vi "校准设置页.vi"() -> ()   [LabVIEW 2016, in "斯坦道总磷.lvlib"]
uses:
  <vilib>/ptbypt/NI_PtbyPt.lvlib
panel:
  in  "校准任务":bool
  in  "历史数据导入":T1(radio)
  out "刷新时间":string
  out "模型刷新":bool
  in  "校准按钮":T1(radio)
  in  "仪器写入":bool
  in  "辅助计算":bool
  in  "曲线模型":T2={"标液浓度1"=0.0, "测量吸光度1"=0.0, "样品1启用"=FALSE, "标液浓度2"=0.0, "测量吸光度2"=0.0, "样品2启用"=FALSE, "标液浓度3"=0.0, "测量吸光度3"=0.0, "样品3启用"=FALSE, "标液浓度4"=0.0, "测量吸光度4"=0.0, "样品4启用"=FALSE, "标液浓度5"=0.0, "测量吸光度5"=0.0, "样品5启用"=FALSE, "模型"=enum."线性", "精度"=4.0, "XY图"=[], "拟合公式"="", "r^2"=0.0, "标样一校准时间"=timestamp(0 s since 1904-01-01), "标样二校准时间"=timestamp(0 s since 1904-01-01), "标样三校准时间"=timestamp(0 s since 1904-01-01), "标样四校准时间"=timestamp(0 s since 1904-01-01), "标样五校准时间"=timestamp(0 s since 1904-01-01), "二次方程"={"c"=0.0, "x"=0.0, "x^2"=0.0}, "标定时间"=timestamp(0 s since 1904-01-01)} {"标定时间" format="%<%y/%m/%d %H:%M:%S>T"; "标样五校准时间" format="%<%y/%m/%d %H:%M:%S>T"; "标样四校准时间" format="%<%y/%m/%d %H:%M:%S>T"; "标样三校准时间" format="%<%y/%m/%d %H:%M:%S>T"; "标样二校准时间" format="%<%y/%m/%d %H:%M:%S>T"; "标样一校准时间" format="%<%y/%m/%d %H:%M:%S>T"; "r^2" format="%.7f"; "测量吸光度5" format="%#.6f"; "测量吸光度4" format="%#.6f"; "测量吸光度3" format="%#.6f"; "测量吸光度2" format="%#.6f"; "测量吸光度1" format="%#.6f"}
  in  "测量模式":T3(ring)
  in  "参数下拉列表":u16(ring)
  in  "量程下拉列表":enum16{"低量程", "高量程"}(ring)
  # "校准时间"
  # "标液浓度"
  # "吸光值"
  # "空白"
  # "标样一"
  # "标样二"
  # "零点"
  # "跨度"
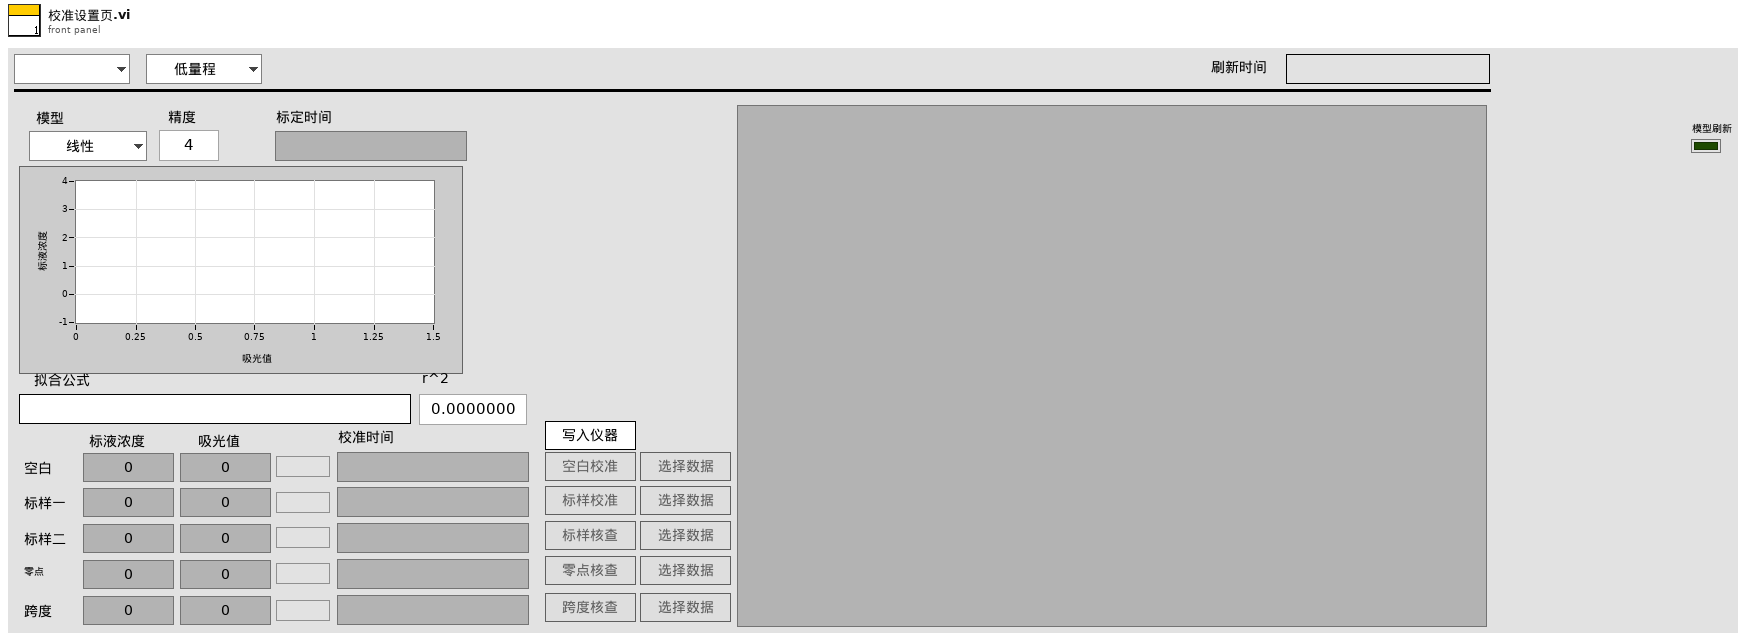
[diagram p1: front panel]
types:
  T1 = enum32{"未选择", "空白校准", "标样校准", "标样核查", "零点核查", "跨度核查"}
  T2 = cluster{"标液浓度1":dbl, "测量吸光度1":dbl, "样品1启用":bool, "标液浓度2":dbl, "测量吸光度2":dbl, "样品2启用":bool, "标液浓度3":dbl, "测量吸光度3":dbl, "样品3启用":bool, "标液浓度4":dbl, "测量吸光度4":dbl, "样品4启用":bool, "标液浓度5":dbl, "测量吸光度5":dbl, "样品5启用":bool, "模型":enum32{"线性", "多项式"}, "精度":dbl, "XY图":cluster{"X Values":dbl[], "Y Values":dbl[]}[], "拟合公式":string, "r^2":dbl, "标样一校准时间":timestamp, "标样二校准时间":timestamp, "标样三校准时间":timestamp, "标样四校准时间":timestamp, "标样五校准时间":timestamp, "二次方程":cluster{"c":dbl, "x":dbl, "x^2":dbl}, "标定时间":timestamp}
  T3 = enum16{"跨度核查", "水样测量", "零点核查", "标样核查", "加标回收", "快捷测试", "空白校准", "标样校准"}
  T4 = typedef "斯坦道总磷.lvlib/校准任务.ctl" = cluster{"id":u16, "任务类型":enum16{"未选择", "空白校准", "标样校准", "标样核查", "零点核查", "跨度核查"}, "量程下拉列表":enum16{"低量程", "高量程"}, "状态":enum16{"已执行", "待执行", "执行中", "停止"}, "标液浓度":dbl, "吸光值":dbl, "校准时间":timestamp}
  T5 = enum8{"Enabled", "Disabled", "Disabled and Grayed Out"}
  T6 = typedef "LVStringsAndValuesArrayTypeDef_U16.ctl" = cluster{"String":string, "Value":u16}[]
  T7 = cluster{"标液浓度1":dbl, "测量吸光度1":dbl, "样品1启用":bool, "标液浓度2":dbl, "测量吸光度2":dbl, "样品2启用":bool, "标液浓度3":dbl, "测量吸光度3":dbl, "样品3启用":bool, "标液浓度4":dbl, "测量吸光度4":dbl, "样品4启用":bool, "标液浓度5":dbl, "测量吸光度5":dbl, "样品5启用":bool, "模型":enum32{"线性", "多项式"}, "精度":dbl, "XY图":cluster{"X Values":dbl[], "Y Values":dbl[]}[], "拟合公式":string, "r^2":dbl, "标样一校准时间":timestamp, "标样二校准时间":timestamp, "标样三校准时间":timestamp, "标样四校准时间":timestamp, "标样五校准时间":timestamp, "二次方程":cluster{"c":dbl, "x":dbl, "x^2":dbl}, "标定时间":timestamp}[]
  T8 = cluster{"时间":timestamp, "标液值":dbl, "检测值":dbl, "吸光值":dbl}
  T9 = enum32{"Bad", "Idle", "Run top level", "Running"}
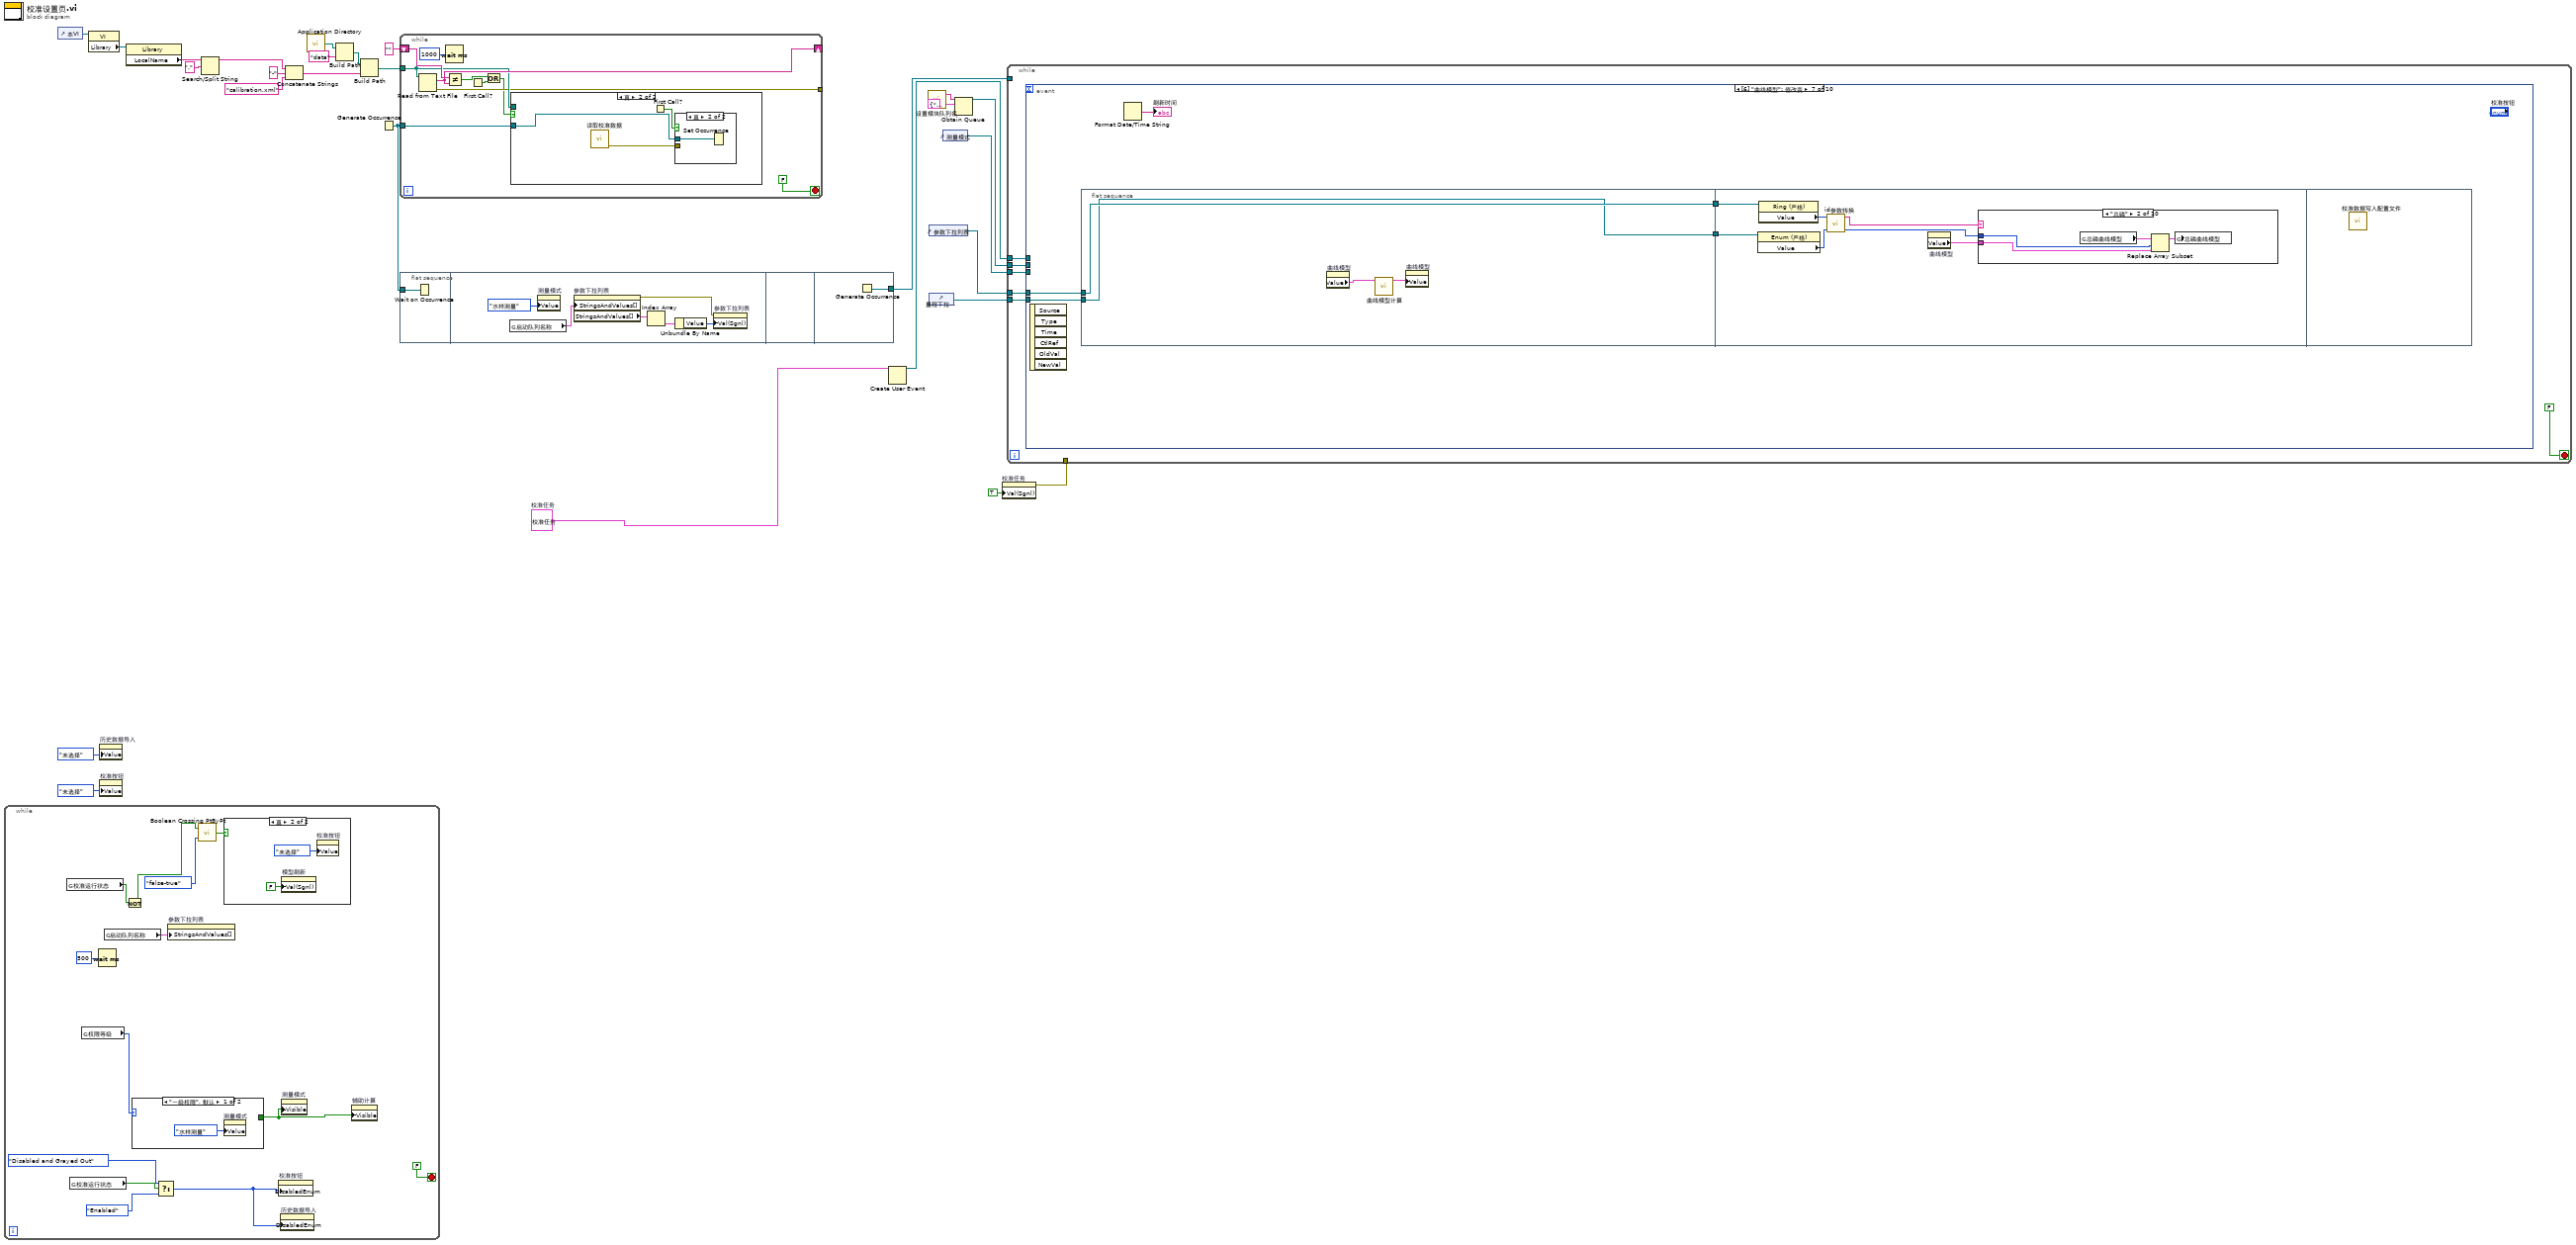
[diagram p0: block diagram]
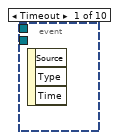
[diagram p4: hidden frame]
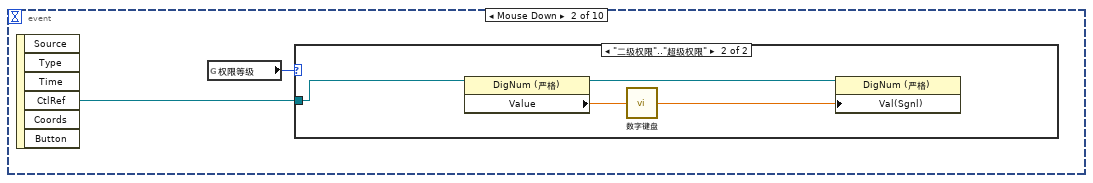
[diagram p5: hidden frame]
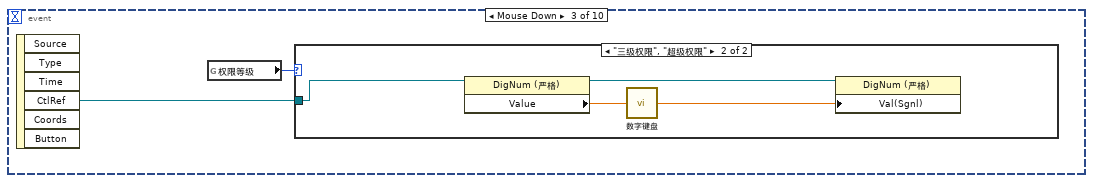
[diagram p7: hidden frame]
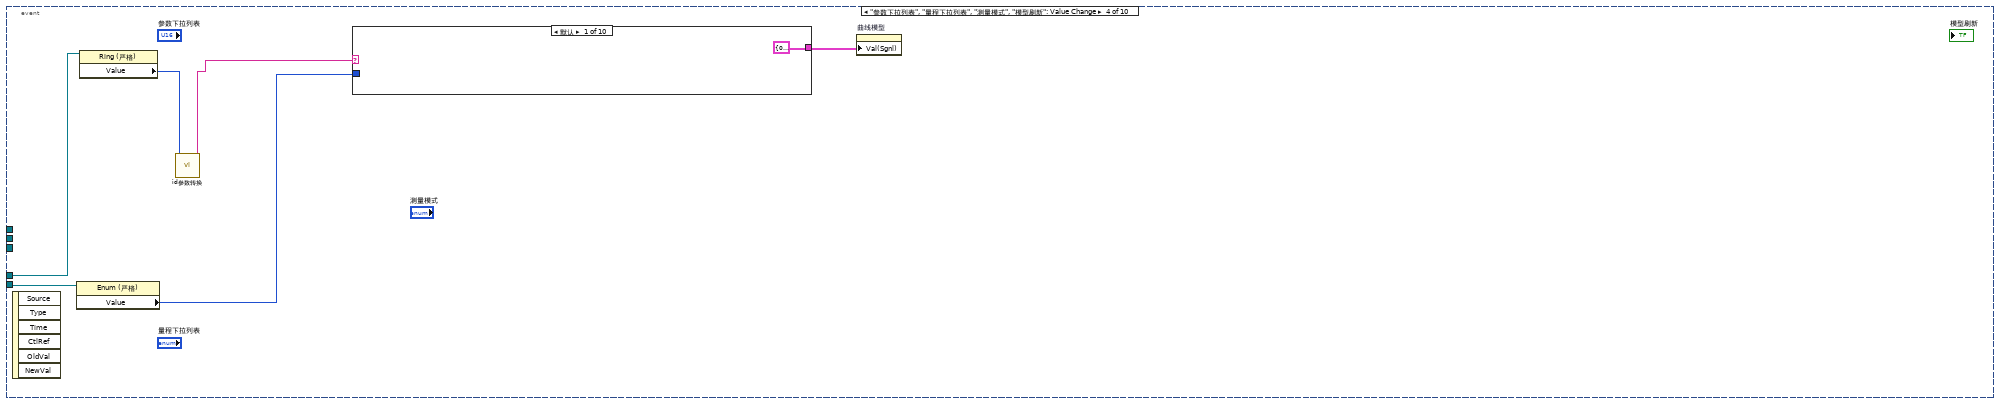
[diagram p9: hidden frame]
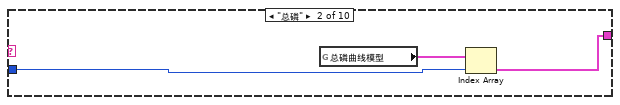
[diagram p10: hidden frame]
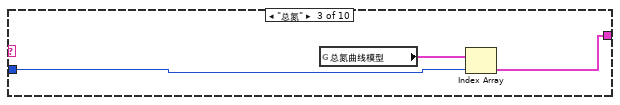
[diagram p11: hidden frame]
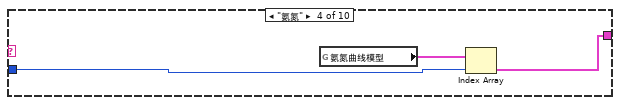
[diagram p12: hidden frame]
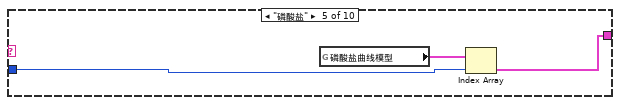
[diagram p13: hidden frame]
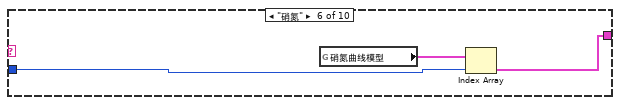
[diagram p14: hidden frame]
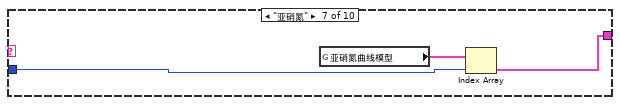
[diagram p15: hidden frame]
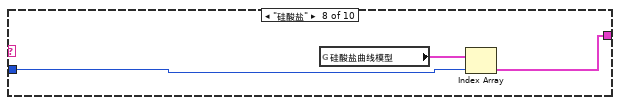
[diagram p16: hidden frame]
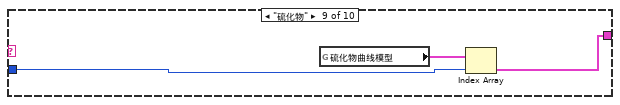
[diagram p17: hidden frame]
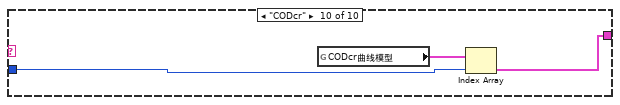
[diagram p18: hidden frame]
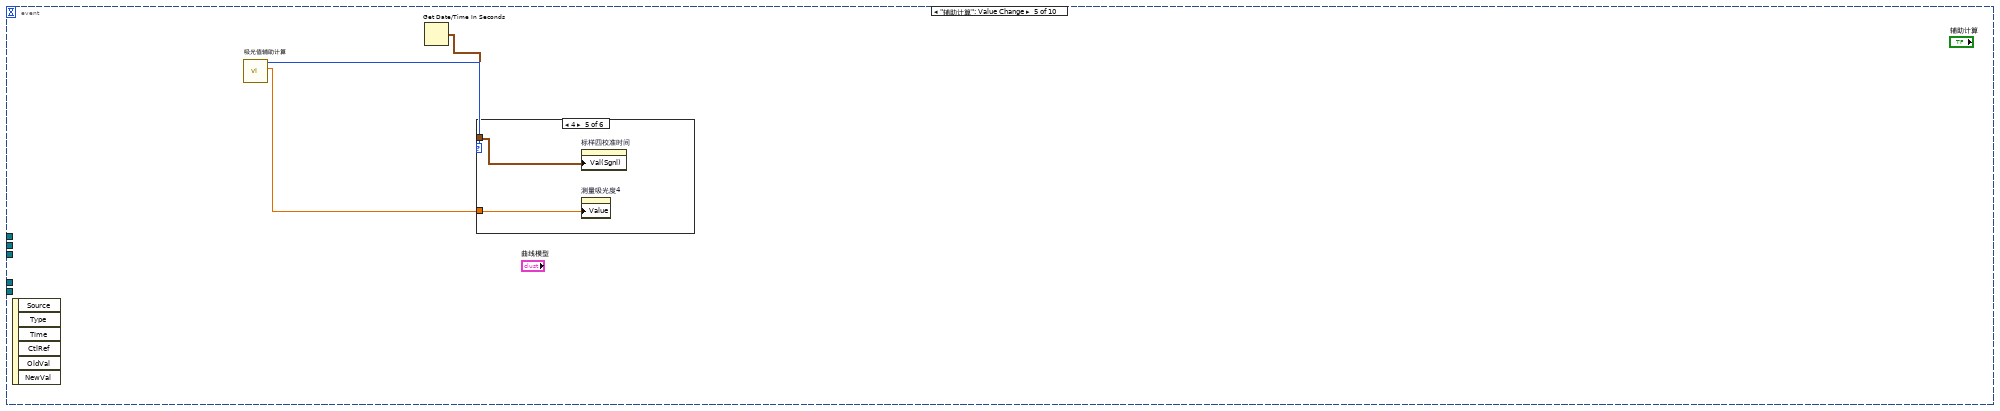
[diagram p19: hidden frame]
diagram:
  w3 = T4 {"id"=1, "任务类型"=enum."未选择", "量程下拉列表"=enum."低量程", "状态"=enum."已执行", "标液浓度"=0.0, "吸光值"=0.0, "校准时间"=timestamp(0 s since 1904-01-01)}  # 校准任务
  n1 = while {
    stop <- FALSE stop-if-true
    n2 = global read "VAR总磷总氮全局变量.vi" "校准运行状态"() -> (w34:bool)
    n3 = global read "VAR总磷总氮全局变量.vi" "校准运行状态"() -> (w31:bool)
    n4 = global read "VAR总磷总氮全局变量.vi" "权限等级"() -> (w38:enum16{"一级权限", "二级权限", "三级权限", "超级权限"})
    n5 = Wait (ms)(milliseconds to wait=u32 500 ("等待时间（毫秒）")) -> ()  [unwired: 1 out]
    n6 = global read "总磷总氮断电保存全局变量.vi" "启动队列名称"() -> (w35:cluster{"String":string, "Value":u16}[])
    n7 = Not(x=w34) -> (.not. x?=w33:bool)
    n8 = case shown="\"一级权限\", 默认" w38 {
      tunnel: [_ TRUE ("可见")] -> w32
      frame "一级权限", Default {
        n9 = property on="测量模式" class="Enum (严格)"("Value"=T3."水样测量" ("测量模式")) -> ()  [unwired: 2 in, 2 out]
      }
      frame "三级权限", "超级权限" {
      }
    }
    n10 = Select(t=T5."Disabled and Grayed Out" ("禁用"), s=w31, f=T5."Enabled" ("禁用")) -> (s? t:f=w29:T5)
    n11 = property on="参数下拉列表" class="Ring (严格)"("StringsAndValues[]"=w35) -> ()  [unwired: 2 in, 2 out]
    n12 = call <vilib>:"Boolean Crossing PtByPt.vi"("direction"=enum16{"either", "false-true", "true-false"}."false-true", "input"=w33) -> ("crossing"=w36:bool)  [unwired: 1 in]
    n13 = case shown="真" w36 {
      frame False {
      }
      frame True {
        n14 = property on="模型刷新" class="Bool (严格)"("Val(Sgnl)"=FALSE ("值(信号)")) -> ()  [unwired: 2 in, 2 out]
        n15 = property on="校准按钮" class="RadioBtnsControl (严格)"("Value"=T1."未选择" ("校准按钮")) -> ()  [unwired: 2 in, 2 out]
      }
    }
    n16 = property on="校准按钮" class="RadioBtnsControl (严格)"("DisabledEnum"=w29) -> ()  [unwired: 2 in, 2 out]
    n17 = property on="历史数据导入" class="RadioBtnsControl (严格)"("DisabledEnum"=w29) -> ()  [unwired: 2 in, 2 out]
    n18 = property on="测量模式" class="Enum (严格)"("Visible"=w32) -> ()  [unwired: 2 in, 2 out]
    n19 = property on="辅助计算" class="Bool"("Visible"=w32) -> ()  [unwired: 2 in, 2 out]
  }
  n20 = control-ref of="本VI"() -> (w15:refnum<vi>)
  n21 = property class="VI"(reference=w15) -> ("Library"=w16:refnum<vi>)  [unwired: 1 in, 2 out]
  n22 = property on="历史数据导入" class="RadioBtnsControl (严格)"("Value"=T1."未选择" ("历史数据导入")) -> ()  [unwired: 2 in, 2 out]
  n23 = property on="校准按钮" class="RadioBtnsControl (严格)"("Value"=T1."未选择" ("校准按钮")) -> ()  [unwired: 2 in, 2 out]
  n24 = property class="Library"(reference=w16) -> ("LocalName"=w13:string)  [unwired: 1 in, 2 out]
  n25 = Search/Split String(string=w13, search string/char (-)="." ("搜索字符串/字符(-)")) -> (substring before match=w11:string)  [unwired: 1 in, 2 out]
  n26 = Concatenate Strings(w11, "-" ("字符串"), "calibration.xml" ("名称或相对路径")) -> (w8:string)
  n27 = call <vilib>:"Application Directory.vi"() -> ("Application Directory"=w17:path)
  n28 = Build Path(base path=w17, name or relative path="data" ("名称或相对路径")) -> (appended path=w14:path)
  n29 = Build Path(base path=w14, name or relative path=w8) -> (appended path=w7:path)
  n30 = Generate Occurrence() -> (w6:refnum<k4>)
  n31 = while {
    shift-right: [w51] -> _
    shift-left: "" -> [w53]
    tunnel: w7 -> [w50]
    tunnel: [w48] -> _
    tunnel: w6 -> [w47]
    stop <- FALSE stop-if-true
    n32 = Read from Text File(file (use dialog)=w50) -> (text=w51:string, error out=w48:errorcluster)  [unwired: 3 in, 2 out]
    n33 = Wait (ms)(milliseconds to wait=u32 1000 ("等待时间（毫秒）")) -> ()  [unwired: 1 out]
    n34 = Not Equal?(x=w53, y=w51) -> (x != y?=w52:bool)
    n35 = First Call?() -> (First Call?: T/F=w45:bool)
    n36 = Or(x=w52, y=w45) -> (x .or. y?=w46:bool)
    n37 = case shown="真" w46 {
      tunnel: w50 -> [_ _]
      tunnel: w47 -> [_ w57]
      frame False {
      }
      frame True {
        n38 = call "读取校准数据.vi"() -> ("错误输出"=w56:errorcluster)  [unwired: 11 in]
        n39 = First Call?() -> (First Call?: T/F=w55:bool)
        n40 = case shown="真" w55 {
          tunnel: w57 -> [_ w58]
          tunnel: w56 -> [_ _]
          frame False {
          }
          frame True {
            n41 = Set Occurrence(w58) -> ()
          }
        }
      }
    }
  }
  n42 = flat-sequence {
    tunnel: w6 -> [w59]
    tunnel: [w66] -> w27
    frame #0 {
      n43 = Wait on Occurrence(2:w59) -> ()  [unwired: 2 in, 1 out]
    }
    frame #1 {
      n44 = global read "总磷总氮断电保存全局变量.vi" "启动队列名称"() -> (w61:cluster{"String":string, "Value":u16}[])
      n45 = property on="测量模式" class="Enum (严格)"("Value"=T3."水样测量" ("测量模式")) -> ()  [unwired: 2 in, 2 out]
      n46 = property on="参数下拉列表" class="Ring (严格)"("StringsAndValues[]"=w61) -> (error out=w64:errorcluster, "StringsAndValues[]"=w62:T6)  [unwired: 2 in, 1 out]
      n47 = Index Array(array=w62) -> (element=w63:cluster{"String":string, "Value":u16})  [unwired: 1 in]
      n48 = Unbundle By Name(w63) -> ("Value"=w65:u16)
      n49 = property on="参数下拉列表" class="Ring (严格)"(error in=w64, "Val(Sgnl)"=w65) -> ()  [unwired: 1 in, 2 out]
    }
    frame #2 {
    }
    frame #3 {
      n50 = Generate Occurrence() -> (w66:refnum<k4>)
    }
  }
  n51 = Create User Event(user event datatype=w3) -> (user event=w4:refnum<user-event>)  [unwired: 1 in, 1 out]
  n52 = call "设置模块队列名.vi"() -> ("Msg"=w25:string)  [unwired: 5 in]
  n53 = control-ref of="参数下拉列表"() -> (w22:refnum<vi>)
  n54 = control-ref of="量程下拉列表"() -> (w20:refnum<vi>)
  n55 = control-ref of="测量模式"() -> (w21:refnum<vi>)
  n56 = Obtain Queue(name (unnamed)=w25, element data type=cluster{"命令":string, "data":variant} {"命令"="", "data"=variant}) -> (queue out=w24:refnum<queue>)  [unwired: 3 in, 2 out]
  n57 = property on="校准任务" class="Bool (严格)"("Val(Sgnl)"=TRUE ("值(信号)")) -> (error out=w2:errorcluster)  [unwired: 2 in, 1 out]
  n58 = while {
    tunnel: w27 -> [_]
    tunnel: w22 -> [w71]
    tunnel: w21 -> [w70]
    tunnel: w20 -> [w69]
    tunnel: w24 -> [w68]
    tunnel: w4 -> [w67]
    tunnel: w2 -> [_]
    stop <- FALSE stop-if-true
    n59 = event shown="[6] \"曲线模型\": 值改变" {
      selector: _ -> [_ _ _ _ _ _ _ _ _ _]
      dyn-events: _ -> [_ _ _ _ _ _ _ _ _ _]
      timeout: _ -> [_ _ _ _ _ _ _ _ _ _]
      tunnel: w71 -> [_ _ _ w89 _ w144 w189 w243 w271 _]
      tunnel: w70 -> [_ _ _ _ _ w142 _ w238 w266 _]
      tunnel: w69 -> [_ _ _ w87 _ w140 w187 w242 w270 _]
      tunnel: w68 -> [_ _ _ _ _ _ _ w244 w272 _]
      tunnel: w67 -> [_ _ _ _ _ _ _ w237 w265 w301]
      event Timeout {
        n60 = event-data() -> ()  [unwired: 1 in, 3 out]
      }
      event "曲线模型.标液浓度1", "曲线模型.标液浓度2", "曲线模型.标液浓度3", "曲线模型.标液浓度4", "曲线模型.标液浓度5", "曲线模型.精度": Mouse Down {
        n61 = event-data() -> ("CtlRef"=w74:refnum<vi>)  [unwired: 1 in, 5 out]
        n62 = global read "VAR总磷总氮全局变量.vi" "权限等级"() -> (w73:enum16{"一级权限", "二级权限", "三级权限", "超级权限"})
        n63 = case shown="\"二级权限\"..\"超级权限\"" w73 {
          tunnel: w74 -> [_ w78]
          frame "一级权限", Default {
          }
          frame "二级权限".."超级权限" {
            n64 = property class="DigNum (严格)"(reference=w78) -> (reference out=w76:refnum<vi>, "Value"=w77:dbl)  [unwired: 1 in, 1 out]
            n65 = call "数字键盘.vi"("OldNumber"=w77) -> ("NewNumber"=w75:dbl)
            n66 = property class="DigNum (严格)"(reference=w76, "Val(Sgnl)"=w75) -> ()  [unwired: 1 in, 2 out]
          }
        }
      }
      event "曲线模型.测量吸光度1", "曲线模型.测量吸光度2", "曲线模型.测量吸光度3", "曲线模型.测量吸光度4", "曲线模型.测量吸光度5": Mouse Down {
        n67 = event-data() -> ("CtlRef"=w80:refnum<vi>)  [unwired: 1 in, 5 out]
        n68 = global read "VAR总磷总氮全局变量.vi" "权限等级"() -> (w79:enum16{"一级权限", "二级权限", "三级权限", "超级权限"})
        n69 = case shown="\"三级权限\", \"超级权限\"" w79 {
          tunnel: w80 -> [_ w84]
          frame "一级权限", Default {
          }
          frame "三级权限", "超级权限" {
            n70 = property class="DigNum (严格)"(reference=w84) -> (reference out=w82:refnum<vi>, "Value"=w83:dbl)  [unwired: 1 in, 1 out]
            n71 = call "数字键盘.vi"("OldNumber"=w83) -> ("NewNumber"=w81:dbl)
            n72 = property class="DigNum (严格)"(reference=w82, "Val(Sgnl)"=w81) -> ()  [unwired: 1 in, 2 out]
          }
        }
      }
      event "参数下拉列表", "量程下拉列表", "测量模式", "模型刷新": Value Change {
        n73 = event-data() -> ()  [unwired: 1 in, 6 out]
        n74 = property class="Enum (严格)"(reference=w87) -> ("Value"=w85:enum16{"低量程", "高量程"})  [unwired: 1 in, 2 out]
        n75 = property class="Ring (严格)"(reference=w89) -> ("Value"=w90:u16)  [unwired: 1 in, 2 out]
        n76 = call "id参数转换.vi"("id"=w90) -> ("table输出"=w88:string)  [unwired: 9 in, 1 out]
        n77 = case shown="默认" w88 {
          tunnel: w85 -> [_ w92 w95 w98 w101 w104 w107 w110 w113 w116]
          tunnel: [T2 {"标液浓度1"=0.0, "测量吸光度1"=0.0, "样品1启用"=FALSE, "标液浓度2"=0.0, "测量吸光度2"=0.0, "样品2启用"=FALSE, "标液浓度3"=0.0, "测量吸光度3"=0.0, "样品3启用"=FALSE, "标液浓度4"=0.0, "测量吸光度4"=0.0, "样品4启用"=FALSE, "标液浓度5"=0.0, "测量吸光度5"=0.0, "样品5启用"=FALSE, "模型"=enum."线性", "精度"=0.0, "XY图"=[], "拟合公式"="", "r^2"=0.0, "标样一校准时间"=timestamp(0 s since 1904-01-01), "标样二校准时间"=timestamp(0 s since 1904-01-01), "标样三校准时间"=timestamp(0 s since 1904-01-01), "标样四校准时间"=timestamp(0 s since 1904-01-01), "标样五校准时间"=timestamp(0 s since 1904-01-01), "二次方程"={"c"=0.0, "x"=0.0, "x^2"=0.0}, "标定时间"=timestamp(0 s since 1904-01-01)} ("总磷曲线模型") w93 w96 w99 w102 w105 w108 w111 w114 w117] -> w86
          frame Default {
          }
          frame "总磷" {
            n78 = global read "校准数据全局变量.vi" "总磷曲线模型"() -> (w94:T7)
            n79 = Index Array(array=w94, index=w92) -> (element=w93:T2)
          }
          frame "总氮" {
            n80 = global read "校准数据全局变量.vi" "总氮曲线模型"() -> (w97:T7)
            n81 = Index Array(array=w97, index=w95) -> (element=w96:T2)
          }
          frame "氨氮" {
            n82 = global read "校准数据全局变量.vi" "氨氮曲线模型"() -> (w100:T7)
            n83 = Index Array(array=w100, index=w98) -> (element=w99:T2)
          }
          frame "磷酸盐" {
            n84 = global read "校准数据全局变量.vi" "磷酸盐曲线模型"() -> (w103:T7)
            n85 = Index Array(array=w103, index=w101) -> (element=w102:T2)
          }
          frame "硝氮" {
            n86 = global read "校准数据全局变量.vi" "硝氮曲线模型"() -> (w106:T7)
            n87 = Index Array(array=w106, index=w104) -> (element=w105:T2)
          }
          frame "亚硝氮" {
            n88 = global read "校准数据全局变量.vi" "亚硝氮曲线模型"() -> (w109:T7)
            n89 = Index Array(array=w109, index=w107) -> (element=w108:T2)
          }
          frame "硅酸盐" {
            n90 = global read "校准数据全局变量.vi" "硅酸盐曲线模型"() -> (w112:T7)
            n91 = Index Array(array=w112, index=w110) -> (element=w111:T2)
          }
          frame "硫化物" {
            n92 = global read "校准数据全局变量.vi" "硫化物曲线模型"() -> (w115:T7)
            n93 = Index Array(array=w115, index=w113) -> (element=w114:T2)
          }
          frame "CODcr" {
            n94 = global read "校准数据全局变量.vi" "CODcr曲线模型"() -> (w118:T7)
            n95 = Index Array(array=w118, index=w116) -> (element=w117:T2)
          }
        }
        n96 = property on="曲线模型" class="Clust (严格)"("Val(Sgnl)"=w86) -> ()  [unwired: 2 in, 2 out]
      }
      event "辅助计算": Value Change {
        n97 = event-data() -> ()  [unwired: 1 in, 6 out]
        n98 = call "吸光值辅助计算.vi"() -> ("X"=w120:dbl, "吸光值导出"=w121:u16)  [unwired: 10 in]
        n99 = Get Date/Time In Seconds() -> (seconds since 1Jan1904=w119:timestamp)
        n100 = case shown="4" w121 {
          tunnel: w120 -> [_ w123 w125 w127 w129 w131]
          tunnel: w119 -> [_ w122 w124 w126 w128 w130]
          frame 0, Default {
          }
          frame 1 {
            n101 = property on="标样一校准时间" class="AbsTime (严格)"("Val(Sgnl)"=w122) -> ()  [unwired: 2 in, 2 out]
            n102 = property on="测量吸光度1" class="DigNum (严格)"("Value"=w123) -> ()  [unwired: 2 in, 2 out]
          }
          frame 2 {
            n103 = property on="标样二校准时间" class="AbsTime (严格)"("Val(Sgnl)"=w124) -> ()  [unwired: 2 in, 2 out]
            n104 = property on="测量吸光度2" class="DigNum (严格)"("Value"=w125) -> ()  [unwired: 2 in, 2 out]
          }
          frame 3 {
            n105 = property on="标样三校准时间" class="AbsTime (严格)"("Val(Sgnl)"=w126) -> ()  [unwired: 2 in, 2 out]
            n106 = property on="测量吸光度3" class="DigNum (严格)"("Value"=w127) -> ()  [unwired: 2 in, 2 out]
          }
          frame 4 {
            n107 = property on="标样四校准时间" class="AbsTime (严格)"("Val(Sgnl)"=w128) -> ()  [unwired: 2 in, 2 out]
            n108 = property on="测量吸光度4" class="DigNum (严格)"("Value"=w129) -> ()  [unwired: 2 in, 2 out]
          }
          frame 5 {
            n109 = property on="标样五校准时间" class="AbsTime (严格)"("Val(Sgnl)"=w130) -> ()  [unwired: 2 in, 2 out]
            n110 = property on="测量吸光度5" class="DigNum (严格)"("Value"=w131) -> ()  [unwired: 2 in, 2 out]
          }
        }
      }
      event "仪器写入": Value Change {
        n111 = event-data() -> ()  [unwired: 1 in, 6 out]
        n112 = property class="Enum (严格)"(reference=w142) -> ("Value"=w141:T3)  [unwired: 1 in, 2 out]
        n113 = property class="Enum (严格)"(reference=w140) -> ("Value"=w139:enum16{"低量程", "高量程"})  [unwired: 1 in, 2 out]
        n114 = property class="Ring (严格)"(reference=w144) -> ("Value"=w143:u16)  [unwired: 1 in, 2 out]
        n115 = property on="二次方程" class="Clust (严格)"() -> ("Value"=w133:cluster{"c":dbl, "x":dbl, "x^2":dbl})  [unwired: 2 in, 2 out]
        n116 = Unbundle By Name(w133) -> ("x^2"=w135:dbl, "x"=w136:dbl, "c"=w137:dbl)
        n117 = Bundle By Name(cluster=cluster{"X^2":dbl, "X":dbl, "b":dbl} {"X^2"=0.0, "X"=0.0, "b"=0.0} ("公式"), "X^2"=w135, "X"=w136, "b"=w137) -> (w132:cluster{"X^2":dbl, "X":dbl, "b":dbl})
        n118 = global read "VAR总磷总氮全局变量.vi" "权限等级"() -> (w138:enum16{"一级权限", "二级权限", "三级权限", "超级权限"})
        n119 = case shown="\"一级权限\", 默认" w138 {
          tunnel: w143 -> [w153 w185]
          tunnel: w141 -> [w152 w184]
          tunnel: w139 -> [w151 w183]
          tunnel: w132 -> [w145 w182]
          frame "一级权限", Default {
            n120 = Cluster To Array(cluster=w145) -> (array=w150:dbl[])
            n121 = Add Array Elements(numeric array=w150) -> (sum=w149:dbl)
            n122 = Equal To 0?(x=w149) -> (x = 0?=w147:bool)
            n123 = Not A Number/Path/Refnum?(number/path/refnum=w149) -> (NaN/Path/Refnum?=w148:bool)
            n124 = Or(x=w147, y=w148) -> (x .or. y?=w146:bool)
            n125 = case shown="假" w146 {
              tunnel: w153 -> [w159 _]
              tunnel: w152 -> [w158 _]
              tunnel: w151 -> [w157 _]
              tunnel: w145 -> [w154 _]
              frame False {
                n126 = Two Button Dialog(message="请再一次确认是否导入" ("消息")) -> (T button?=w155:bool)  [unwired: 2 in]
                n127 = case shown="真" w155 {
                  tunnel: w159 -> [_ w161]
                  tunnel: w158 -> [_ w167]
                  tunnel: w157 -> [_ w160]
                  tunnel: w154 -> [_ w162]
                  frame False {
                  }
                  frame True {
                    n128 = for {
                      N: 8 -> [_]
                      tunnel: w161 -> [w173]
                      tunnel: w167 -> [_]
                      tunnel: w160 -> [w172]
                      shift-right: [w171] -> w165
                      shift-left: errorcluster {"status"=FALSE, "code"=0, "source"=""} ("error out") -> [w168]
                      tunnel: w162 -> [w169]
                      i -> [w170]
                      n129 = call "总磷总氮公式写入.vi"("公式"=w169, "error in (no error)"=w168, "量程"=w172, "测量模式"=w170, "测量参数"=w173) -> ("error out"=w171:errorcluster)  [unwired: 6 in]
                    }
                    n130 = case shown="无错误" w165 {
                      tunnel: ["写入成功" "写入失败"] -> w166
                      tunnel: w161 -> [w177 _]
                      tunnel: w160 -> [w176 _]
                      frame No Error {
                        n131 = Get Date/Time In Seconds() -> (seconds since 1Jan1904=w178:timestamp)
                        n132 = property on="标定时间" class="AbsTime (严格)"("Val(Sgnl)"=w178) -> (error out=w174:errorcluster)  [unwired: 2 in, 1 out]
                        n133 = property on="曲线模型" class="Clust (严格)"(error in=w174) -> ("Value"=w175:T2)  [unwired: 1 in, 2 out]
                        n134 = call "校准记录.vi"("曲线模型"=w175, "量程"=w176, "校准参数"=w177) -> ()  [unwired: 8 in, 1 out]
                      }
                      frame Error {
                      }
                    }
                    n135 = One Button Dialog(message=w166) -> ()  [unwired: 1 in, 1 out]
                  }
                }
              }
              frame True {
                n136 = One Button Dialog(message="校准数据异常，请重新校准！" ("消息")) -> ()  [unwired: 1 in, 1 out]
              }
            }
          }
          frame "三级权限", "超级权限" {
            n137 = call "公式复合写入.vi"("公式"=w182, "量程下拉列表"=w183, "测量模式"=w184, "参数下拉列表"=w185) -> ()  [unwired: 8 in]
          }
        }
      }
      event "曲线模型": Value Change {
        n138 = event-data() -> ()  [unwired: 1 in, 6 out]
        n139 = flat-sequence {
          tunnel: [w194] -> w190
          tunnel: w189 -> [w194]
          tunnel: [w193] -> w188
          tunnel: w187 -> [w193]
          tunnel: w190 -> [w200]
          tunnel: w188 -> [w197]
          frame #0 {
            n140 = property on="曲线模型" class="Clust (严格)"() -> ("Value"=w192:T2)  [unwired: 2 in, 2 out]
            n141 = call "曲线模型计算.vi"("曲线模型"=w192) -> ("输出簇"=w191:T2)  [unwired: 10 in]
            n142 = property on="曲线模型" class="Clust (严格)"("Value"=w191) -> ()  [unwired: 2 in, 2 out]
          }
          frame #1 {
            n143 = property class="Enum (严格)"(reference=w197) -> ("Value"=w196:enum16{"低量程", "高量程"})  [unwired: 1 in, 2 out]
            n144 = property class="Ring (严格)"(reference=w200) -> ("Value"=w199:u16)  [unwired: 1 in, 2 out]
            n145 = call "id参数转换.vi"("id"=w199) -> ("table输出"=w198:string)  [unwired: 9 in, 1 out]
            n146 = property on="曲线模型" class="Clust (严格)"() -> ("Value"=w195:T2)  [unwired: 2 in, 2 out]
            n147 = case shown="\"总磷\"" w198 {
              tunnel: w195 -> [_ w202 w208 w211 w214 w218 w222 w226 w230 w235]
              tunnel: w196 -> [_ w201 w205 w209 w213 w217 w221 w225 w229 w233]
              frame Default {
              }
              frame "总磷" {
                n148 = global read "校准数据全局变量.vi" "总磷曲线模型"() -> (w203:T7)
                n149 = Replace Array Subset(array=w203, new element=w202, index=w201) -> (w204:T7)
                n150 = global write "校准数据全局变量.vi" "总磷曲线模型"(w204) -> ()
              }
              frame "总氮" {
                n151 = global read "校准数据全局变量.vi" "总氮曲线模型"() -> (w207:T7)
                n152 = Replace Array Subset(array=w207, new element=w208, index=w205) -> (w206:T7)
                n153 = global write "校准数据全局变量.vi" "总氮曲线模型"(w206) -> ()
              }
              frame "氨氮" {
                n154 = global read "校准数据全局变量.vi" "氨氮曲线模型"() -> (w212:T7)
                n155 = Replace Array Subset(array=w212, new element=w211, index=w209) -> (w210:T7)
                n156 = global write "校准数据全局变量.vi" "氨氮曲线模型"(w210) -> ()
              }
              frame "磷酸盐" {
                n157 = global read "校准数据全局变量.vi" "磷酸盐曲线模型"() -> (w216:T7)
                n158 = Replace Array Subset(array=w216, new element=w214, index=w213) -> (w215:T7)
                n159 = global write "校准数据全局变量.vi" "磷酸盐曲线模型"(w215) -> ()
              }
              frame "硝氮" {
                n160 = global read "校准数据全局变量.vi" "硝氮曲线模型"() -> (w220:T7)
                n161 = Replace Array Subset(array=w220, new element=w218, index=w217) -> (w219:T7)
                n162 = global write "校准数据全局变量.vi" "硝氮曲线模型"(w219) -> ()
              }
              frame "亚硝氮" {
                n163 = global read "校准数据全局变量.vi" "亚硝氮曲线模型"() -> (w224:T7)
                n164 = Replace Array Subset(array=w224, new element=w222, index=w221) -> (w223:T7)
                n165 = global write "校准数据全局变量.vi" "亚硝氮曲线模型"(w223) -> ()
              }
              frame "硅酸盐" {
                n166 = global read "校准数据全局变量.vi" "硅酸盐曲线模型"() -> (w228:T7)
                n167 = Replace Array Subset(array=w228, new element=w226, index=w225) -> (w227:T7)
                n168 = global write "校准数据全局变量.vi" "硅酸盐曲线模型"(w227) -> ()
              }
              frame "硫化物" {
                n169 = global read "校准数据全局变量.vi" "硫化物曲线模型"() -> (w232:T7)
                n170 = Replace Array Subset(array=w232, new element=w230, index=w229) -> (w231:T7)
                n171 = global write "校准数据全局变量.vi" "硫化物曲线模型"(w231) -> ()
              }
              frame "CODcr" {
                n172 = global read "校准数据全局变量.vi" "CODcr曲线模型"() -> (w236:T7)
                n173 = Replace Array Subset(array=w236, new element=w235, index=w233) -> (w234:T7)
                n174 = global write "校准数据全局变量.vi" "CODcr曲线模型"(w234) -> ()
              }
            }
          }
          frame #2 {
            n175 = call "校准数据写入配置文件.vi"() -> ()  [unwired: 11 in, 1 out]
          }
        }
        n176 = Format Date/Time String() -> (date/time string=→"刷新时间":string)  [unwired: 3 in]
      }
      event "校准按钮": Value Change {
        n177 = event-data() -> ("NewVal"=w239:T1)  [unwired: 1 in, 5 out]
        n178 = Not Equal?(x=w239, y=T1."未选择") -> (x != y?=w240:bool)
        n179 = case shown="真" w240 {
          tunnel: w244 -> [_ _]
          tunnel: w243 -> [_ w254]
          tunnel: w242 -> [_ w253]
          tunnel: w239 -> [_ w249]
          tunnel: w238 -> [_ _]
          tunnel: w237 -> [_ w252]
          frame False {
          }
          frame True {
            w246 = T4 {"id"=1, "任务类型"=enum."未选择", "量程下拉列表"=enum."低量程", "状态"=enum."待执行", "标液浓度"=0.0, "吸光值"=0.0, "校准时间"=timestamp(0 s since 1904-01-01)}  # 校准任务
            n180 = property on="曲线模型" class="Clust (严格)"() -> ("Value"=w248:T2)  [unwired: 2 in, 2 out]
            n181 = case shown="\"未选择\", 默认" w249 {
              tunnel: w248 -> [_ w256 w258 w260 w262 w264]
              tunnel: [_ w255 w257 w259 w261 w263] -> w247
              frame "未选择", Default {
              }
              frame "空白校准" {
                n182 = Unbundle By Name(w256) -> ("标液浓度1"=w255:dbl)
              }
              frame "标样校准" {
                n183 = Unbundle By Name(w258) -> ("标液浓度2"=w257:dbl)
              }
              frame "标样核查" {
                n184 = Unbundle By Name(w260) -> ("标液浓度3"=w259:dbl)
              }
              frame "零点核查" {
                n185 = Unbundle By Name(w262) -> ("标液浓度4"=w261:dbl)
              }
              frame "跨度核查" {
                n186 = Unbundle By Name(w264) -> ("标液浓度5"=w263:dbl)
              }
            }
            n187 = property class="Enum (严格)"(reference=w253) -> ("Value"=w250:enum16{"低量程", "高量程"})  [unwired: 1 in, 2 out]
            n188 = property class="Ring (严格)"(reference=w254) -> ("Value"=w251:u16)  [unwired: 1 in, 2 out]
            n189 = Bundle By Name(cluster=w246, "id"=w251, "任务类型"=w249, "量程下拉列表"=w250, "标液浓度"=w247) -> (w245:T4)
            n190 = Generate User Event(user event=w252, event data cluster=w245) -> ()  [unwired: 2 in, 2 out]
          }
        }
      }
      event "历史数据导入": Value Change {
        n191 = event-data() -> ("NewVal"=w267:T1)  [unwired: 1 in, 5 out]
        n192 = Not Equal?(x=w267, y=T1."未选择") -> (x != y?=w268:bool)
        n193 = case shown="真" w268 {
          tunnel: w272 -> [_ _]
          tunnel: w271 -> [_ w283]
          tunnel: w270 -> [_ w274]
          tunnel: w267 -> [_ w282]
          tunnel: w266 -> [_ _]
          tunnel: w265 -> [_ w276]
          frame False {
          }
          frame True {
            n194 = case shown="\"跨度核查\"" w282 {
              tunnel: [T3."水样测量" ("测量模式") T3."空白校准" ("测量模式") T3."标样校准" ("测量模式") T3."标样核查" ("测量模式") T3."零点核查" ("测量模式") T3."跨度核查" ("测量模式")] -> w280
              frame "未选择", Default {
              }
              frame "空白校准" {
              }
              frame "标样校准" {
              }
              frame "标样核查" {
              }
              frame "零点核查" {
              }
              frame "跨度核查" {
              }
            }
            n195 = property class="Enum (严格)"(reference=w274) -> ("Value"=w273:enum16{"低量程", "高量程"})  [unwired: 1 in, 2 out]
            n196 = property class="Ring (严格)"(reference=w283) -> ("Value"=w275:u16)  [unwired: 1 in, 2 out]
            n197 = property on="历史数据导入" class="RadioBtnsControl (严格)"("Value"=T1."未选择" ("历史数据导入")) -> ()  [unwired: 2 in, 2 out]
            n198 = call "id参数转换.vi"("id"=w275) -> ("table输出"=w281:string)  [unwired: 9 in, 1 out]
            n199 = call "校准数据选择表.vi"("测量模式"=w280, "table"=w281) -> ("布尔"=w279:bool, "输出"=w278:T8)  [unwired: 8 in]
            n200 = case shown="真" w279 {
              tunnel: w278 -> [_ w291]
              tunnel: w282 -> [_ w293]
              tunnel: w276 -> [_ w292]
              tunnel: w275 -> [_ w290]
              tunnel: w273 -> [_ w289]
              frame False {
              }
              frame True {
                w287 = T4 {"id"=1, "任务类型"=enum."未选择", "量程下拉列表"=enum."低量程", "状态"=enum."已执行", "标液浓度"=0.0, "吸光值"=0.0, "校准时间"=timestamp(0 s since 1904-01-01)}  # 校准任务
                n201 = Unbundle By Name(w291) -> ("标液值"=w284:dbl, "吸光值"=w285:dbl, "时间"=w286:timestamp)
                n202 = Bundle By Name(cluster=w287, "id"=w290, "任务类型"=w293, "量程下拉列表"=w289, "标液浓度"=w284, "吸光值"=w285, "校准时间"=w286) -> (w288:T4)
                n203 = Generate User Event(user event=w292, event data cluster=w288) -> ()  [unwired: 2 in, 2 out]
              }
            }
          }
        }
      }
      event "校准任务": Value Change {
        n204 = event-data() -> ("NewVal"=w300:bool)  [unwired: 1 in, 5 out]
        n205 = invoke on="子面板" class="SubPnl" method="Remove VI"() -> (error out=w302:errorcluster)  [unwired: 3 in, 2 out]
        n206 = case shown="真" w300 {
          tunnel: w302 -> [_ w309]
          tunnel: w301 -> [_ w306]
          frame False {
          }
          frame True {
            n207 = vi-ref "校准任务设置.vi"() -> (w308:refnum<vi>)
            n208 = property class="VI"(reference=w308) -> (reference out=w304:refnum<vi>, "Name"=w307:string, "Exec.State"=w305:T9)  [unwired: 1 in, 1 out]
            n209 = case shown="\"Idle\"" w305 {
              tunnel: w307 -> [_ w321]
              tunnel: w306 -> [_ w318]
              tunnel: [w310 w314] -> w303
              tunnel: w304 -> [w310 w314]
              frame "Bad", Default {
              }
              frame "Idle" {
                n210 = property on="模型" class="Enum (严格)"() -> ("Value"=w312:enum32{"线性", "多项式"})  [unwired: 2 in, 2 out]
                n211 = Open VI Reference(type specifier VI Refnum (for type only)=refnum<vi> refnum, vi path=w321, options=128 ("选项")) -> (vi reference=w319:refnum<vi>, error out=w316:errorcluster)  [unwired: 3 in]
                n212 = property on="精度" class="DigNum (严格)"() -> ("Value"=w311:dbl)  [unwired: 2 in, 2 out]
                n213 = call-by-ref "开始异步调用"(reference=w319, error in=w316, "精度"=w311, "模型"=w312, "用户事件"=w318) -> (reference out=w317:refnum<vi>, error out=w315:errorcluster)  [unwired: 9 in]
                n214 = Close Reference(reference=w317, error in (no error)=w315) -> ()  [unwired: 1 out]
              }
            }
            n215 = invoke on="子面板" class="SubPnl" method="Insert VI"(error in=w309, "VI Ref"=w303) -> ()  [unwired: 2 in, 4 out]
          }
        }
      }
    }
  }
